vi "Test.vi"(8 "error in (no error)":errorcluster, 10 "board image":T1, 11 "Board Design in":refnum<class "Board Design.lvclass">) -> (0 "error out":errorcluster, 2 "pass?":T2, 3 "Test name":string)   [LabVIEW 2018, in "Board Design.lvclass"]
doc: "Image check for blocks that are common to all types of boards."
uses:
  Board Design.lvclass
  Common/Pass Fail Boolean.ctl
  Common/Board Image.ctl
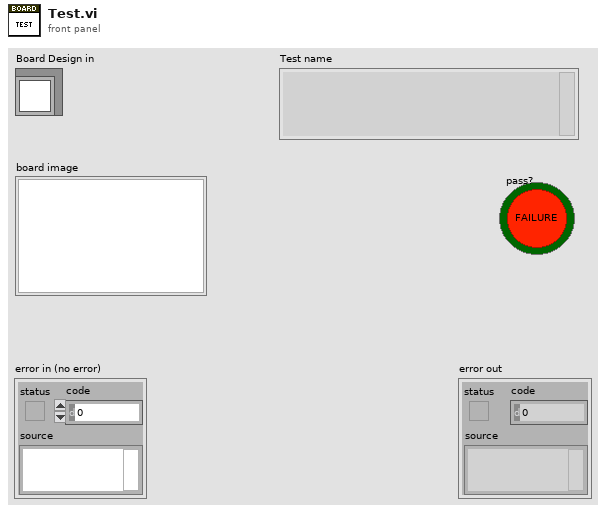
[diagram p1: front panel]
types:
  T1 = typedef "Board Image.ctl" = picture
  T2 = typedef "Pass Fail Boolean.ctl" = bool
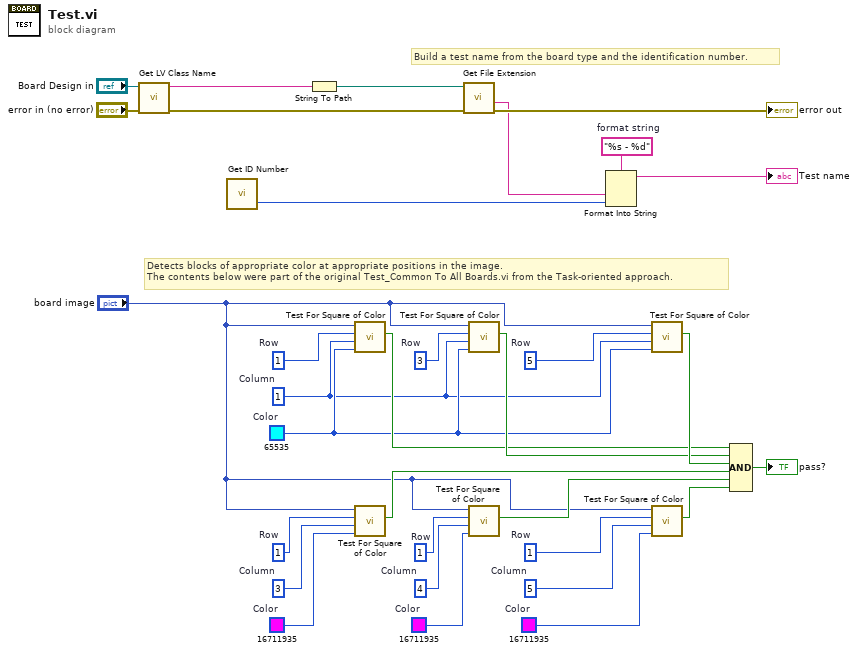
[diagram p0: block diagram]
diagram:
  w4 = "%s - %d"  # format string
  w19 = i16 5  # Column
  w20 = i16 1  # Row
  w18 = u32 16711935  # Color
  w16 = i16 4  # Column
  w15 = i16 1  # Row
  w17 = u32 16711935  # Color
  w13 = i16 3  # Column
  w14 = i16 1  # Row
  w12 = u32 16711935  # Color
  w9 = i16 5  # Row
  w8 = i16 3  # Row
  w10 = i16 1  # Column
  w7 = i16 1  # Row
  w11 = u32 65535  # Color
  # "Build a test name from the board type and the identification number."
  # "Detects blocks of appropriate color at appropriate positions in the image.\nThe contents below were part of the original Test_Common To All Boards.vi from the Task-oriented approach."
  n1 = call <vilib>:"Get LV Class Name.vi"("error in (no error)"="error in (no error)", "object"="Board Design in") -> ("error out"=w29:errorcluster, "class name"=w30:string)  [unwired: 8 in]
  n2 = call "Get ID Number.vi"() -> ("id number"=w2:u32)  [unwired: 2 in]
  n3 = String To Path(string=w30) -> (path=w31:path)
  n4 = call "Test For Square of Color.vi"("color"=w11, "column"=w10, "row"=w7, "board image"="board image") -> ("pass?"=w21:T2)  [unwired: 7 in]
  n5 = call "Test For Square of Color.vi"("color"=w12, "column"=w13, "row"=w14, "board image"="board image") -> ("pass?"=w24:T2)  [unwired: 7 in]
  n6 = call <vilib>:"Get File Extension.vi"("error in (no error)"=w29, "file"=w31) -> ("error out"=→"error out":errorcluster, "filename without extension"=w3:string)  [unwired: 5 in, 3 out]
  n7 = call "Test For Square of Color.vi"("color"=w11, "column"=w10, "row"=w8, "board image"="board image") -> ("pass?"=w22:T2)  [unwired: 7 in]
  n8 = call "Test For Square of Color.vi"("color"=w17, "column"=w16, "row"=w15, "board image"="board image") -> ("pass?"=w25:T2)  [unwired: 7 in]
  n9 = Format Into String(format string=w4, w3, w2) -> (resulting string=→"Test name":string)  [unwired: 2 in, 1 out]
  n10 = call "Test For Square of Color.vi"("color"=w11, "column"=w10, "row"=w9, "board image"="board image") -> ("pass?"=w23:T2)  [unwired: 7 in]
  n11 = call "Test For Square of Color.vi"("color"=w18, "column"=w19, "row"=w20, "board image"="board image") -> ("pass?"=w26:T2)  [unwired: 7 in]
  n12 = Compound Arithmetic op=AND(w21, w22, w23, w24, w25, w26) -> (→"pass?":T2)
